vi "F020_din_get.vi"(8 "error in":errorcluster, 10 "Cluster":cluster{"ADDRESS":u8, "DIG_CH":u8}={"ADDRESS"=170, "DIG_CH"=0} {"ADDRESS" format="%.0x"}, 11 "COM in":string="COM4") -> (0 "error out":errorcluster={"status"=TRUE, "code"=-1073807343, "source"=""}, 1 "Dig State(bool)":bool, 2 "Dig State(num)":u16, 3 "COM out":string="COM4")   [LabVIEW 2016]
doc: "This example performs a serial port write and a serial port read. The parameters set for the serial port must match the parameters of the connected instrument or device. The VISA Configure Serial Port VI sets the configuration parameters. The front panel displays the controls used to configure the basic parameters, such as baud rate, data bits, and parity. The VI passes the VISA resource name to other VIs that perform operations on that VISA resource. The VISA Write function sends a command to the serial device and the VISA Read function returns data based on the command. The VISA Close function then closes the reference to the serial device. It is important to close the reference; otherwise, further communication through that port might not be possible."
panel:
  out "packet ( <xxAABBCC..>":string="<03AA1301>"
  out "Response {xx}":string="{0FFF}"
  # "loopback: <xxAABB>\nwr_dout:   <xxAA11aabbccdd> aa=ch, bb=val, ccdd=timeout[sec]\nrd_ain:      <xxAA13aa> -> {qqww}"
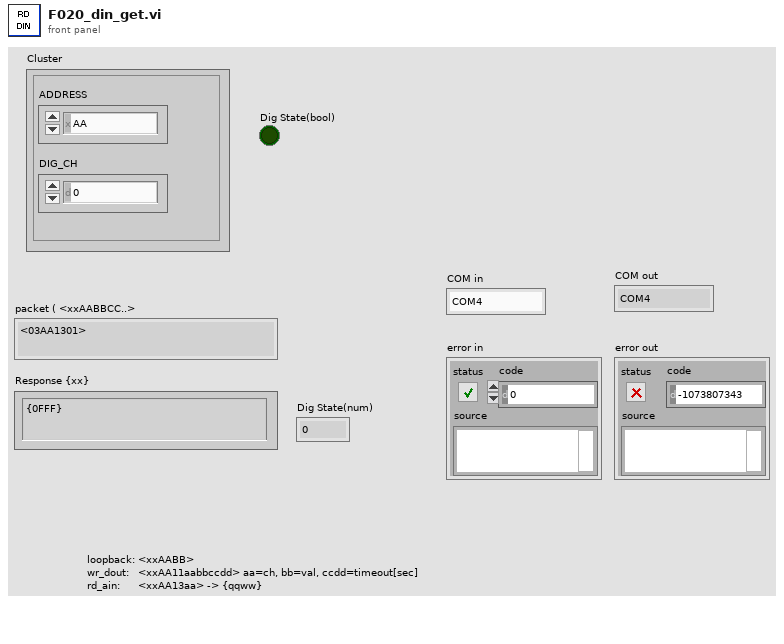
[diagram p1: front panel]
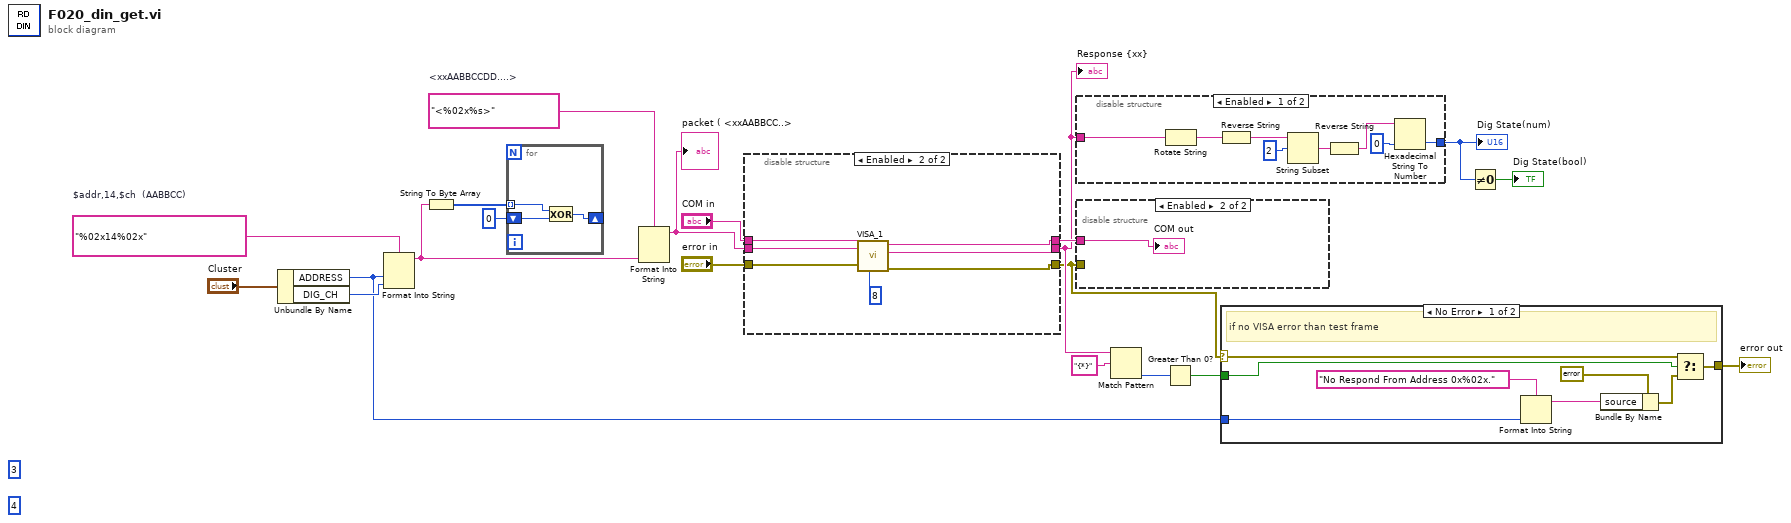
[diagram p0: block diagram]
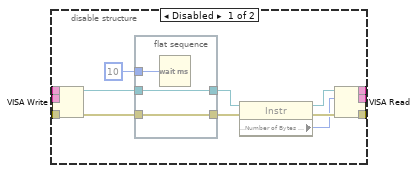
[diagram p2: hidden frame]
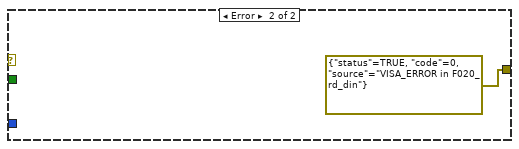
[diagram p3: hidden frame]
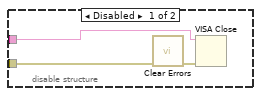
[diagram p4: hidden frame]
diagram:
  (unwired) u32 4 ("delay before read (ms)")
  (unwired) u32 3 ("delay before read (ms)")
  w15 = "%02x14%02x"  # $addr,14,$ch  (AABBCC)
  w10 = "<%02x%s>"  # <xxAABBCCDD....>
  n1 = Unbundle By Name("Cluster") -> ("ADDRESS"=w4:u8, "DIG_CH"=w12:u8)
  n2 = Format Into String(format string=w15, w4, w12) -> (resulting string=w14:string)  [unwired: 2 in, 1 out]
  n3 = String To Byte Array(string=w14) -> (unsigned byte array=w17:u8[])
  n4 = for {
    tunnel: w17 -> [w23] mode=indexing
    shift-right: [w22] -> _
    shift-left: u8 0 -> [w21]
    n5 = Exclusive Or(1:w21, 2:w23) -> (0:w22:u8)
  }
  n6 = Format Into String(format string=w10, w14) -> (resulting string=w11:string)  [unwired: 3 in, 1 out]
  "packet ( <xxAABBCC..>" <- w11
  n7 = disable-structure shown="Enabled" {
    disable-tunnel: [w37 w46] -> w20
    disable-tunnel: "error in" -> [w36 w43]
    disable-tunnel: "COM in" -> [w35 w47]
    disable-tunnel: w11 -> [w26 w45]
    disable-tunnel: [w25 w44] -> w6
    disable-tunnel: [w24 w42] -> w5
    frame Disabled {
      n8 = VISA Write(VISA resource name=w35, write buffer=w26, error in (no error)=w36) -> (VISA resource name out=w32:refnum<visa-resource-name>, error out=w34:errorcluster)  [unwired: 1 out]
      n9 = flat-sequence {
        tunnel: w34 -> [w39]
        tunnel: [w39] -> w33
        tunnel: w32 -> [w38]
        tunnel: [w38] -> w31
        tunnel: u32 10 ("delay before read (ms)") -> [w40]
        frame #0 {
          n10 = Wait (ms)(milliseconds to wait=w40) -> ()  [unwired: 1 out]
        }
      }
      n11 = property class="Instr"(reference=w31, error in=w33) -> (reference out=w29:refnum<visa-resource-name>, error out=w28:errorcluster, "Serial Settings:Number of Bytes at Serial Port"=w27:u32)
      n12 = VISA Read(VISA resource name=w29, byte count=w27, error in (no error)=w28) -> (VISA resource name out=w37:refnum<visa-resource-name>, read buffer=w25:string, error out=w24:errorcluster)  [unwired: 1 out]
    }
    frame Enabled {
      n13 = call "VISA_1.vi"("delay[ms]"=u32 8, "error in"=w43, "wr_buf"=w45, "COM in"=w47) -> ("error out"=w42:errorcluster, "rx_buf"=w44:string, "COM out"=w46:string)  [unwired: 5 in]
    }
  }
  "Response {xx}" <- w6
  n14 = disable-structure shown="Enabled" {
    disable-tunnel: w6 -> [w49 _]
    disable-tunnel: [w48 _] -> w2
    frame Enabled {
      n15 = Rotate String(1:w49) -> (0:w50:string)
      n16 = Reverse String(1:w50) -> (0:w51:string)
      n17 = String Subset(string=w51, offset (0)=2) -> (substring=w53:string)  [unwired: 1 in]
      n18 = Reverse String(1:w53) -> (0:w55:string)
      n19 = Hexadecimal String To Number(string=w55, default (0uL)=u16 0 ("default (0 U32)")) -> (number=w48:u16)  [unwired: 1 in, 1 out]
    }
    frame Disabled {
    }
  }
  "Dig State(num)" <- w2
  n20 = disable-structure shown="Enabled" {
    disable-tunnel: w5 -> [w58 _]
    disable-tunnel: w20 -> [w57 w59]
    frame Disabled {
      n21 = call <vilib>:"Clear Errors.vi"("error in (no error)"=w58) -> ("error out"=w56:errorcluster)  [unwired: 5 in, 1 out]
      n22 = VISA Close(VISA resource name=w57, error in (no error)=w56) -> ()  [unwired: 1 out]
    }
    frame Enabled {
      "COM out" <- w59
    }
  }
  n23 = Match Pattern(string=w6, regular expression="{*}") -> (offset past match=w7:i32)  [unwired: 1 in, 3 out]
  n24 = Greater Than 0?(x=w7) -> (x > 0?=w8:bool)
  n25 = case shown="No Error" w5 {
    selector: w5 -> [w65 _]
    tunnel: w8 -> [w67 _]
    tunnel: [w66 errorcluster {"status"=TRUE, "code"=0, "source"="VISA_ERROR in F020_rd_din"} ("f")] -> w3
    tunnel: w4 -> [w60 _]
    frame No Error {
      # "if no VISA error than test frame"
      n26 = Format Into String(format string="No Respond From Address 0x%02x.", w60) -> (resulting string=w61:string)  [unwired: 2 in, 1 out]
      n27 = Bundle By Name(cluster=errorcluster {"status"=TRUE, "code"=-1, "source"="frameTest ERROR! HW_wr_dout__GP.vi"} ("f"), "source"=w61) -> (w63:errorcluster)
      n28 = Select(t=w65, s=w67, f=w63) -> (s? t:f=w66:errorcluster)
    }
    frame Error {
    }
  }
  "error out" <- w3
  n29 = Not Equal To 0?(x=w2) -> (x != 0?=→"Dig State(bool)":bool)
